vi "UsrProfiles-Update users list.vi"(8 "error in":errorcluster) -> (0 "error out":errorcluster, 3 "Users listbox":refnum<vi>)   [LabVIEW 2017]
uses:
  Globals/gl_UsrProfiles globals.vi
  Global Variables/General Globals.vi
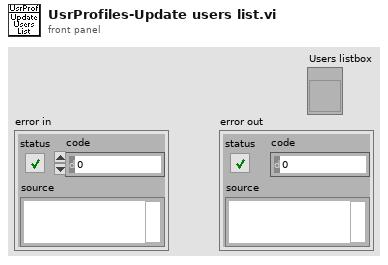
[diagram p1: front panel]
types:
  T1 = typedef "User login window refs.ctl" = cluster{"User profiles window ref":refnum<k9>, "Users listbox":refnum<vi>, "Profiles listbox":refnum<vi>, "Last used":refnum<vi>}
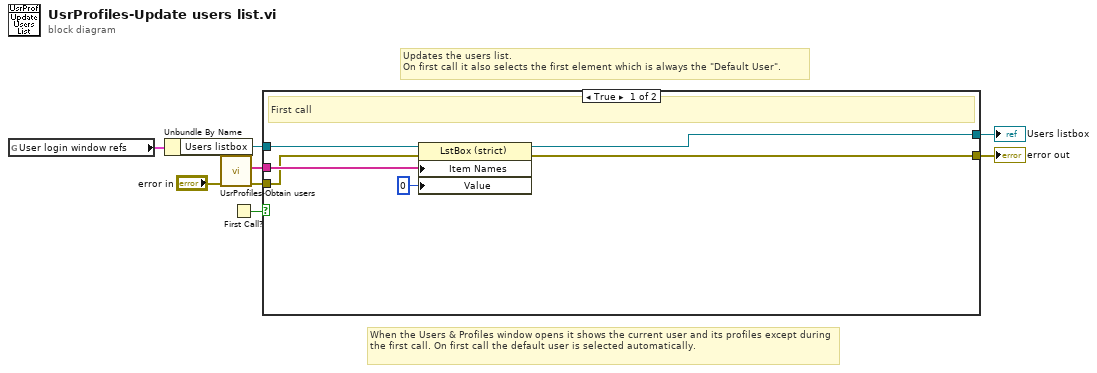
[diagram p0: block diagram]
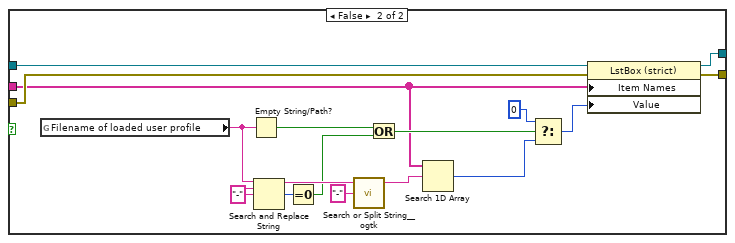
[diagram p2: hidden frame]
diagram:
  # "When the Users & Profiles window opens it shows the current user and its profiles except during the first call. On first call the default user is selected automatically."
  # "Updates the users list.\nOn first call it also selects the first element which is always the \"Default User\"."
  n1 = global read "gl_UsrProfiles globals.vi" "User login window refs"() -> (w7:T1)
  n2 = Unbundle By Name(w7) -> ("Users listbox"=w8:refnum<vi>)
  n3 = call "UsrProfiles-Obtain users.vi"("error in"="error in") -> ("error out"=w6:errorcluster, "User names"=w3:string[])  [unwired: 9 in]
  n4 = First Call?() -> (First Call?: T/F=w2:bool)
  n5 = case shown="True" w2 {
    tunnel: w3 -> [w14 w16]
    tunnel: w8 -> [w13 w31]
    tunnel: [w11 w30] -> w4
    tunnel: w6 -> [w10 w29]
    tunnel: [w9 w15] -> w1
    frame True {
      # "First call"
      n6 = property on="Property Node" class="LstBox (strict)"(reference=w13, error in=w10, "Item Names"=w14, "Value"=0) -> (reference out=w9:refnum<vi>, error out=w11:errorcluster)
    }
    frame False {
      w20 = "-" ("search string/char (-)")
      n7 = global read "General Globals.vi" "Filename of loaded user profile"() -> (w19:string)
      n8 = Empty String/Path?(string/path=w19) -> (empty?=w22:bool)
      n9 = Search and Replace String(input string=w19, search string=w20, replace string=w20) -> (result string=w25:string, number of replacements=w21:i32)  [unwired: 5 in, 2 out]
      n10 = Equal To 0?(x=w21) -> (x = 0?=w24:bool)
      n11 = call <userlib>:"Search or Split String__ogtk.vi"("search string/char (-)"="-", "string"=w25) -> ("substring before match"=w27:string)  [unwired: 1 in, 2 out]
      n12 = Or(x=w22, y=w24) -> (x .or. y?=w23:bool)
      n13 = Search 1D Array(1D array=w16, element=w27) -> (index of element=w28:i32)  [unwired: 1 in]
      n14 = Select(t=0 ("Value"), s=w23, f=w28) -> (s? t:f=w18:i32)
      n15 = property on="Property Node" class="LstBox (strict)"(reference=w31, error in=w29, "Item Names"=w16, "Value"=w18) -> (reference out=w15:refnum<vi>, error out=w30:errorcluster)
    }
  }
  "error out" <- w4
  "Users listbox" <- w1
